vi "题目4.vi"() -> ()   [LabVIEW 2017]
uses:
  <vilib>/Analysis/2dsp.llb/Real FFT.vi
  <vilib>/Analysis/NI_AALPro.lvlib
  <vilib>/measure/NI_MABase.lvlib
panel:
  in  "sampling info 3":cluster{"Fs":dbl, "#s":dbl}={"Fs"=1000.0, "#s"=1000.0} caption="采样信息3" {"Fs" format="%.2p"}
  in  "sampling info 2":cluster{"Fs":dbl, "#s":dbl}={"Fs"=1000.0, "#s"=1000.0} caption="采样信息2" {"Fs" format="%.2p"}
  in  "sampling info":cluster{"Fs":dbl, "#s":dbl}={"Fs"=1000.0, "#s"=1000.0} caption="采样信息1" {"Fs" format="%.2p"}
  in  "amplitude 3":dbl=1.0 caption="幅值3" format="%0.2p"
  in  "frequency 3":dbl=10.0 caption="频率2" format="%0.2p"
  in  "amplitude 2":dbl=1.0 caption="幅值1" format="%0.2p"
  in  "frequency 2":dbl=10.0 caption="频率3" format="%0.2p"
  in  "amplitude":dbl=1.0 caption="幅值2" format="%0.2p"
  in  "frequency":dbl=10.0 caption="频率1" format="%0.2p"
  out "频域信号":dbl[](graph)
  out "时域信号":dbl[](graph)
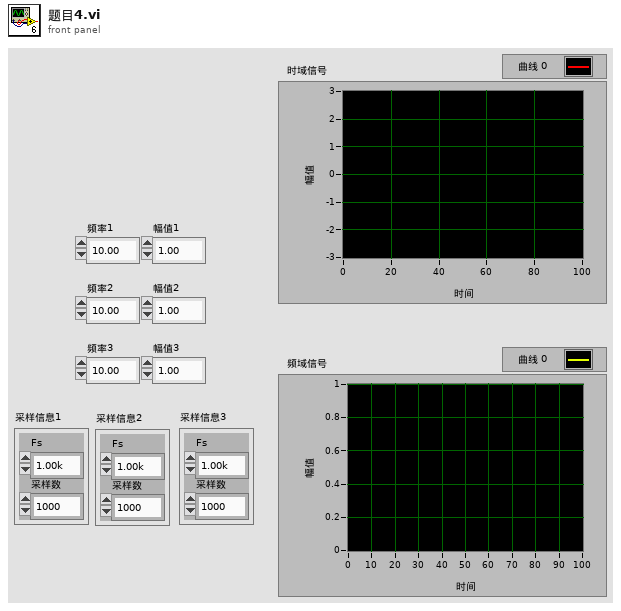
[diagram p1: front panel]
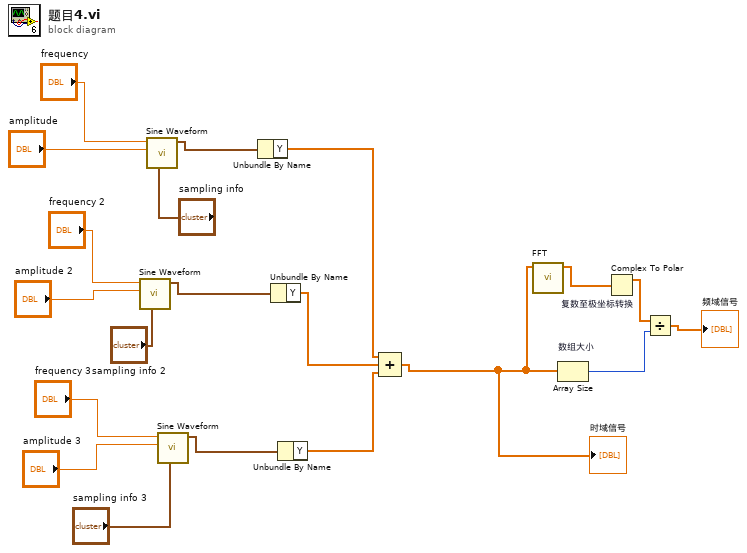
[diagram p0: block diagram]
diagram:
  n1 = call <vilib>:"Sine Waveform.vi"("sampling info"="sampling info 2", "amplitude"="amplitude 2", "frequency"="frequency 2") -> ("signal out"=w15:waveform(dbl))  [unwired: 7 in, 1 out]
  n2 = call <vilib>:"Sine Waveform.vi"("sampling info"="sampling info", "amplitude"="amplitude", "frequency"="frequency") -> ("signal out"=w16:waveform(dbl))  [unwired: 7 in, 1 out]
  n3 = call <vilib>:"Sine Waveform.vi"("sampling info"="sampling info 3", "amplitude"="amplitude 3", "frequency"="frequency 3") -> ("signal out"=w14:waveform(dbl))  [unwired: 7 in, 1 out]
  n4 = Unbundle By Name(w16) -> ("Y"=w7:dbl[])
  n5 = Unbundle By Name(w15) -> ("Y"=w6:dbl[])
  n6 = Unbundle By Name(w14) -> ("Y"=w5:dbl[])
  n7 = Compound Arithmetic op=ADD ("复合运算")(w7, w6, w5) -> (w4:dbl[])
  "时域信号" <- w4
  n8 = call-poly <vilib>:"FFT.vi"("X"=w4) -> ("FFT {X}"=w20:cdb[])  [unwired: 9 in, 1 out]
  n9 = Array Size "数组大小"(array=w4) -> (size(s)=w17:i32)
  n10 = Complex To Polar "复数至极坐标转换"(r * e^(i*theta)=w20) -> (r=w19:dbl[])  [unwired: 1 out]
  n11 = Divide(x=w19, y=w17) -> (x/y=→"频域信号":dbl[])
